vi "Init FPs.vi"(8 "error in (no error)":errorcluster, 11 "GUI View in":refnum<class "GUI View.lvclass">) -> (0 "error out":errorcluster, 3 "GUI View out":refnum<class "GUI View.lvclass">)   [LabVIEW 2023, in "GUI Views.lvlib" / "GUI View.lvclass"]
uses:
  GUI View.lvclass
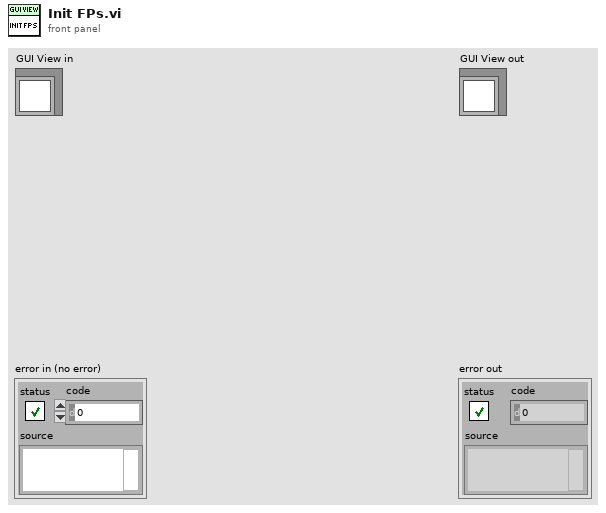
[diagram p1: front panel]
types:
  T1 = enum32{"Invalid", "Standard", "Closed", "Hidden", "Minimized", "Maximized"}
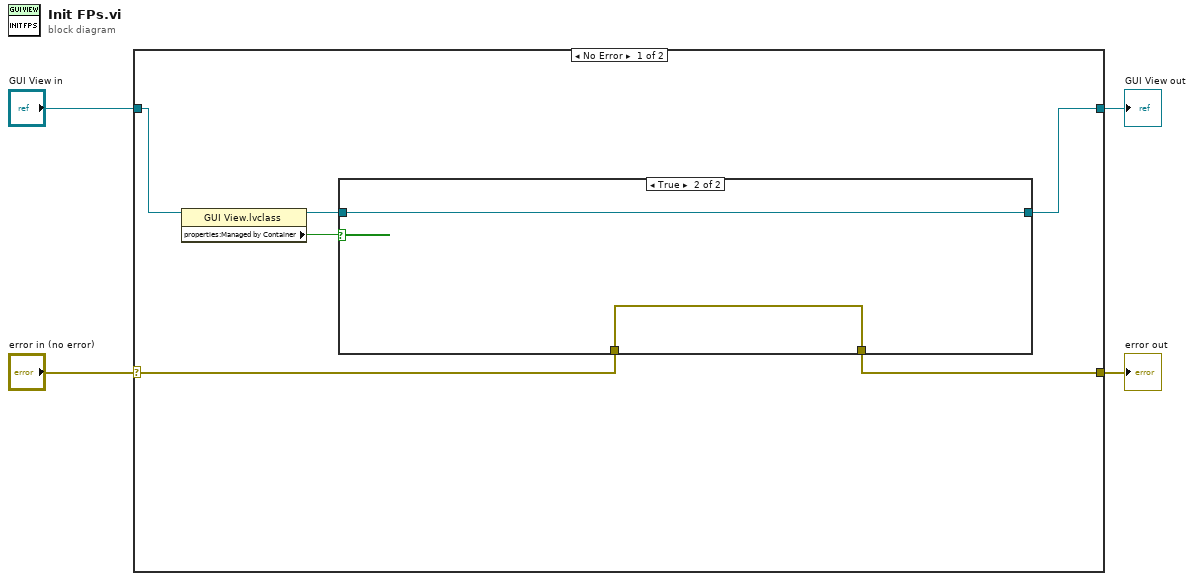
[diagram p0: block diagram]
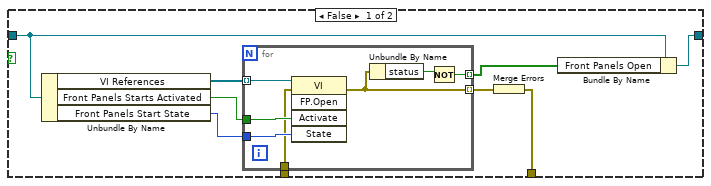
[diagram p2: hidden frame]
diagram:
  n1 = case shown="No Error" "error in (no error)" {
    selector: "error in (no error)" -> [w10 w30]
    tunnel: [w9 w30] -> w3
    tunnel: [w5 w29] -> w1
    tunnel: "GUI View in" -> [w6 w29]
    frame No Error {
      n2 = property class="GUI View.lvclass"(reference=w6) -> (reference out=w7:refnum<class "GUI View.lvclass">, "properties:Managed by Container"=w8:bool)  [unwired: 1 in, 1 out]
      n3 = case shown="True" w8 {
        tunnel: w10 -> [w16 w27]
        tunnel: [w14 w27] -> w9
        tunnel: w7 -> [w13 w28]
        tunnel: [w12 w28] -> w5
        frame False {
          n4 = Unbundle By Name(w13) -> ("VI References"=w19:refnum<vi>[], "Front Panels Starts Activated"=w18:bool, "Front Panels Start State"=w17:T1)
          n5 = for {
            tunnel: w19 -> [w26] mode=indexing
            tunnel: w18 -> [w25]
            tunnel: w17 -> [w24]
            tunnel: w16 -> [w23]
            tunnel: [w22] -> w15 mode=indexing
            tunnel: [w20] -> w11 mode=indexing
            n6 = invoke class="VI" method="FP.Open"(reference=w26, error in=w23, "Activate"=w25, "State"=w24) -> (error out=w22:errorcluster)  [unwired: 1 in, 4 out]
            n7 = Unbundle By Name(w22) -> ("status"=w21:bool)
            n8 = Not(x=w21) -> (.not. x?=w20:bool)
          }
          n9 = Merge Errors(w15) -> (w14:errorcluster)
          n10 = Bundle By Name(cluster=w13, "Front Panels Open"=w11) -> (w12:refnum<class "GUI View.lvclass">)
        }
        frame True {
        }
      }
    }
    frame Error {
    }
  }
  "error out" <- w3
  "GUI View out" <- w1
